vi "Close.vi"(8 "error in":errorcluster, 11 "Fgen PXI CFG in":refnum<class "Fgen PXI CFG.lvclass">) -> (0 "error out":errorcluster, 3 "Fgen PXI CFG out":refnum<class "Fgen PXI CFG.lvclass">)   [LabVIEW 2023, in "HAL.lvlib" / "Fgen PXI.lvlib" / "Fgen PXI CFG.lvclass"]
uses:
  Fgen PXI CFG.lvclass
  Fgen PXI CFG.lvclass/Fgen PXI CFG.ctl
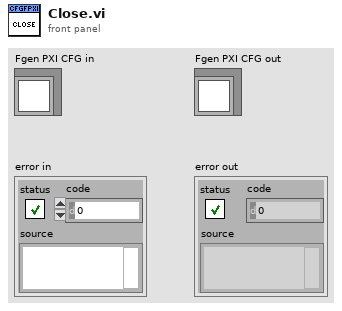
[diagram p1: front panel]
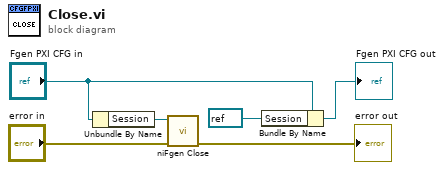
[diagram p0: block diagram]
diagram:
  n1 = Unbundle By Name("Fgen PXI CFG in") -> ("Session"=w6:refnum<k15>)
  n2 = call <instrlib>:"niFgen Close.vi"("error in (no error)"="error in", "Instrument Handle"=w6) -> ("error out"=→"error out":errorcluster)  [unwired: 9 in]
  n3 = Bundle By Name(cluster="Fgen PXI CFG in", "Session"=refnum<k15> refnum) -> (→"Fgen PXI CFG out":refnum<class "Fgen PXI CFG.lvclass">)
